vi "Get Manifold Channel.vi"(8 "error in (no error)":errorcluster, 10 "Manifold Channel":u32, 11 "Gantry Class in":refnum<class "Gantry Class.lvclass">) -> (0 "error out":errorcluster, 2 "On/Off":bool, 3 "Gantry Class out":refnum<class "Gantry Class.lvclass">)   [LabVIEW 2011, in "Gantry Class.lvclass"]
uses:
  Gantry Class.lvclass
  WorkTable Class/WorkTable Class.lvclass
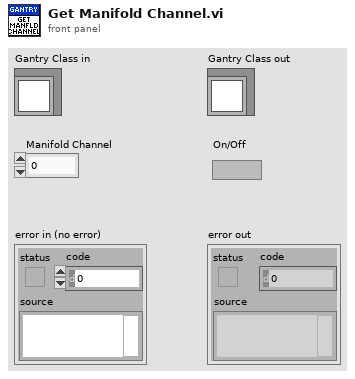
[diagram p1: front panel]
types:
  T1 = typedef "Worktable_Manifold Channel.ctl" = cluster{"Enabled":bool, "Hardware Path":string}
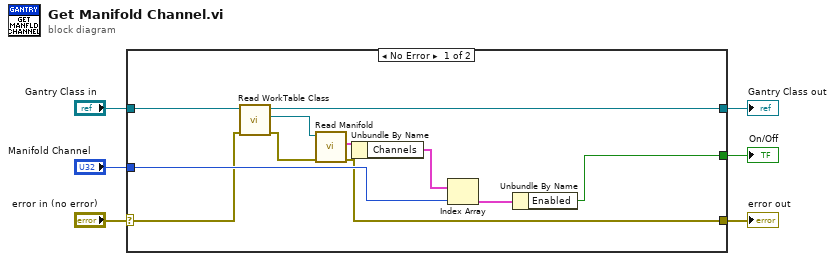
[diagram p0: block diagram]
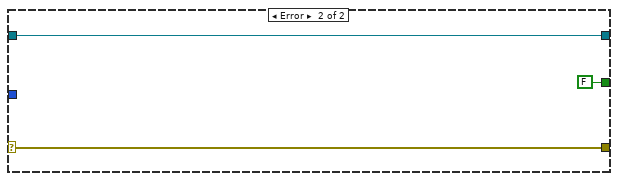
[diagram p2: hidden frame]
diagram:
  n1 = case shown="No Error" "error in (no error)" {
    selector: "error in (no error)" -> [w8 w20]
    tunnel: [w7 w20] -> w5
    tunnel: [w16 w19] -> w3
    tunnel: "Gantry Class in" -> [w17 w19]
    tunnel: "Manifold Channel" -> [w11 _]
    tunnel: [w9 FALSE ("Enabled")] -> w1
    frame No Error {
      n2 = call-dynamic "Read WorkTable Class.vi"("error in"=w8, "Gantry Class in"=w17) -> ("error out"=w14:errorcluster, "WorkTable Class.lvclass"=w15:refnum<class "WorkTable Class.lvclass">, "Gantry Class out"=w16:refnum<class "Gantry Class.lvclass">)  [unwired: 7 in]
      n3 = call-dynamic "Read Manifold.vi"("error in (no error)"=w14, "WorkTable Class in"=w15) -> ("error out"=w7:errorcluster, "Manifold"=w13:cluster{"Channels":T1[]})  [unwired: 7 in, 1 out]
      n4 = Unbundle By Name(w13) -> ("Channels"=w12:T1[])
      n5 = Index Array(array=w12, index=w11) -> (element=w10:T1)
      n6 = Unbundle By Name(w10) -> ("Enabled"=w9:bool)
    }
    frame Error {
    }
  }
  "error out" <- w5
  "Gantry Class out" <- w3
  "On/Off" <- w1
